vi "校准基准_自校端指令.vi"(8 "error in (no error)":errorcluster, 10 "进口":i32, 11 "命令":refnum<queue>) -> (0 "error out":errorcluster)   [LabVIEW 2011]
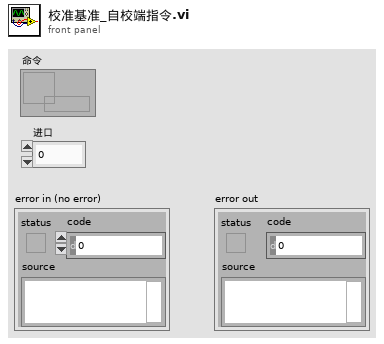
[diagram p1: front panel]
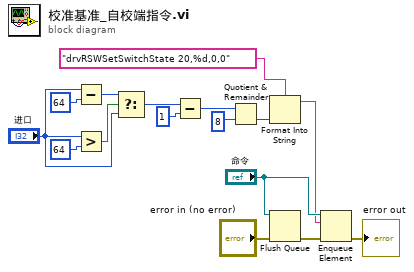
[diagram p0: block diagram]
diagram:
  n1 = Subtract(x="进口", y=64) -> (x-y=w5:i32)
  n2 = Greater?(x="进口", y=64) -> (0:w7:bool)
  n3 = Select(t=w5, s=w7, f="进口") -> (s? t:f=w4:i32)
  n4 = Subtract(x=w4, y=1) -> (x-y=w13:i32)
  n5 = Quotient & Remainder(x=w13, y=8) -> (floor(x/y)=w16:i32)  [unwired: 1 out]
  n6 = Format Into String(format string="drvRSWSetSwitchState 20,%d,0,0" ("格式字符串"), w16) -> (resulting string=w9:string)  [unwired: 2 in, 1 out]
  n7 = Flush Queue(queue="命令", error in (no error)="error in (no error)") -> (error out=w11:errorcluster)  [unwired: 2 out]
  n8 = Enqueue Element(queue="命令", element=w9, error in (no error)=w11) -> (error out=→"error out":errorcluster)  [unwired: 1 in, 2 out]
